vi "module-09-analog-limit.vi"() -> ()   [LabVIEW 2019]
uses:
  samples-common-library/Ctrl_Training_Library_Protected/CtrlTrainingLibary_Protected.lvlib
panel:
  in  "Tab Control":enum32{"Control Panel", "Logic"}(tab)
  out "High Selected":dbl
  in  "Lo Limit":dbl(slide)=-39.370078740157474 min=-100.0 max=100.0 scale=-100.0..100.0
  in  "Input":dbl(slide)=10.0 scale=-100.0..100.0
  out "Low Selected":dbl
  out "Trend":T1(graph)
  in  "Hi Limit":dbl(slide)=40.94488188976379 min=-100.0 max=100.0 scale=-100.0..100.0
  out "High Low Limited":dbl
  out "High Select":dbl(slide)=-39.370078740157474 min=-100.0 max=100.0 scale=-100.0..100.0
  out "Low Select":dbl(slide)=-39.370078740157474 min=-100.0 max=100.0 scale=-100.0..100.0
  out "Hi/Low Limit":dbl(slide)=-39.370078740157474 min=-100.0 max=100.0 scale=-100.0..100.0
  # "High / Low Limit, High / Low Select Test"
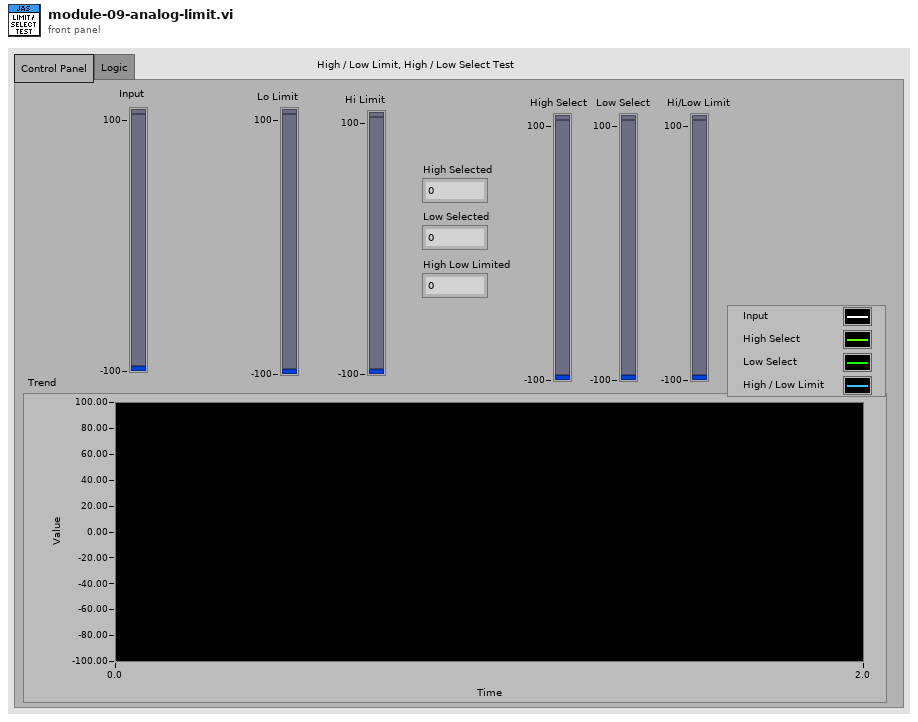
[diagram p1: front panel]
types:
  T1 = cluster{"Input":dbl, "Output":dbl, "Output":dbl, "Output":dbl}
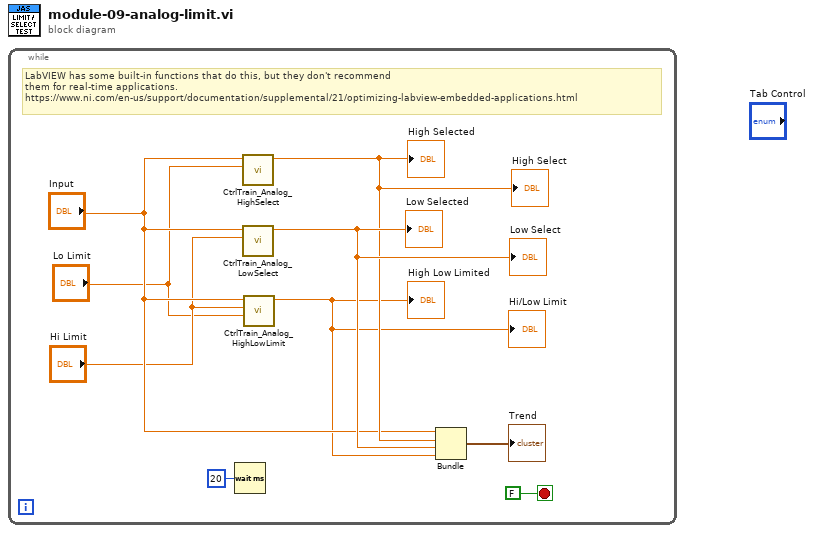
[diagram p0: block diagram]
diagram:
  n1 = while {
    stop <- FALSE stop-if-true
    # "LabVIEW has some built-in functions that do this, but they don't recommend\nthem for real-time applications.\nhttps://www.ni.com/en-us/support/documentation/supplemental/21/optimizing-labview-embedded-applications.html"
    n2 = Wait (ms)(milliseconds to wait=u32 20) -> ()  [unwired: 1 out]
    n3 = call "CtrlTrain_Analog_HighSelect.vi"("Input_2"="Lo Limit", "Input_1"="Input") -> ("Output"=w5:dbl)  [unwired: 9 in]
    "High Selected" <- w5
    "High Select" <- w5
    n4 = call "CtrlTrain_Analog_LowSelect.vi"("Input_2"="Hi Limit", "Input_1"="Input") -> ("Output"=w6:dbl)  [unwired: 9 in]
    "Low Selected" <- w6
    "Low Select" <- w6
    n5 = call "CtrlTrain_Analog_HighLowLimit.vi"("Lo_Limit"="Lo Limit", "Hi_Limit"="Hi Limit", "Input"="Input") -> ("Output"=w1:dbl)  [unwired: 8 in]
    "High Low Limited" <- w1
    "Hi/Low Limit" <- w1
    n6 = Bundle("Input"="Input", "Output"=w5, "Output"=w6, "Output"=w1) -> (→"Trend":T1)  [unwired: 1 in]
  }
